vi "remote.Read Dev.Commands.vi"(8 "error in (no error)":errorcluster, 11 "SLSC Remote in":refnum<class "SLSC Remote.lvclass">) -> (0 "error out":errorcluster, 2 "Dev.Commands":refnum<k21>[](array[refnum]), 3 "SLSC Remote out":refnum<class "SLSC Remote.lvclass">)   [LabVIEW 2016, in "SLSC Interfaces.lvlib" / "SLSC Remote.lvclass"]
uses:
  SLSC Remote.lvclass
  <vilib>/NI/JSON Support for LabVIEW/JSON Data Classes/JSON Helper/JSON Helper.lvclass
  <vilib>/NI/JSON Support for LabVIEW/JSON Data Classes/JSON Array/JSON Array.lvclass
  <vilib>/NI/JSON Support for LabVIEW/JSON Data Classes/JSON Array/Index Array (String Value).vi
  <vilib>/NI/JSON Support for LabVIEW/JSON Data Classes/JSON Helper/To More Specific Type (Array).vi
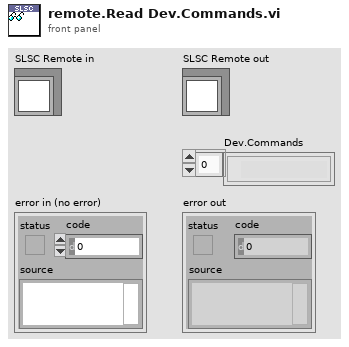
[diagram p1: front panel]
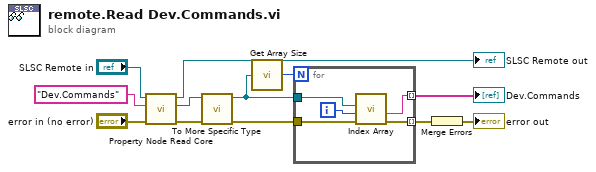
[diagram p0: block diagram]
diagram:
  n1 = call "Property Node Read Core.vi"("error in (no error)"="error in (no error)", "property"="Dev.Commands", "SLSC Remote in"="SLSC Remote in") -> ("error out"=w4:errorcluster, "value"=w8:refnum<class "JSON Null.lvclass">, "SLSC Remote out"=→"SLSC Remote out":refnum<class "SLSC Remote.lvclass">)  [unwired: 6 in]
  n2 = call-poly <vilib>:"To More Specific Type.vi"("error in (no error)"=w4, "JSON Datatype in"=w8) -> ("error out"=w3:errorcluster, "JSON Datatype out"=w6:refnum<class "JSON Array.lvclass">)  [unwired: 8 in]
  n3 = call <vilib>:"Get Array Size.vi"("JSON Array in"=w6) -> ("size(s)"=w7:i32)
  n4 = for {
    N: w7 -> [_]
    tunnel: w6 -> [w17]
    tunnel: [w15] -> w5 mode=indexing
    tunnel: w3 -> [w14]
    tunnel: [w13] -> w2 mode=indexing
    i -> [w16]
    n5 = call-poly <vilib>:"Index Array.vi"("error in (no error)"=w14, "index"=w16, "JSON Array in"=w17) -> ("error out"=w13:errorcluster, "String"=w15:string)  [unwired: 7 in]
  }
  "Dev.Commands" <- w5
  n6 = Merge Errors(w2) -> (→"error out":errorcluster)
